vi "Detect_Level.vi"(8 "High Range":T2, 9 "Low Range":T1, 10 "EncoderDevRef":T3={"DevStatus"={"status"=FALSE, "code"=0, "source"=""}, "EncoderIndex"=enum."Invalid", "CounterIndex"=enum."Ctr 1", "DistancePerCount"=2.0, "Decoding Type"=enum."4x"}) -> (2 "Level":dbl)   [LabVIEW 2014]
uses:
  <vilib>/Rock Robotics/WPI/Encoder/WPI_EncoderDevRef.ctl
  <vilib>/Rock Robotics/SystemInterfaces/Encoder/FPGA_EncoderIdx.ctl
  <vilib>/Rock Robotics/SystemInterfaces/Counter/FPGA_CounterCtrSystemIndex.ctl
  <vilib>/Rock Robotics/WPI/Encoder/WPI_EncoderType.ctl
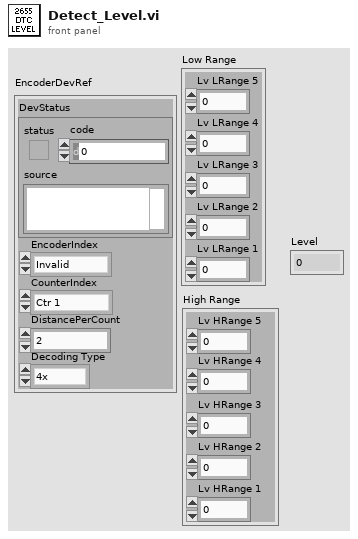
[diagram p1: front panel]
types:
  T1 = cluster{"Lv LRange 1":dbl, "Lv LRange 2":dbl, "Lv LRange 3":dbl, "Lv LRange 4":dbl, "Lv LRange 5":dbl}
  T2 = cluster{"Lv HRange 5":dbl, "Lv HRange 4":dbl, "Lv HRange 3":dbl, "Lv HRange 2":dbl, "Lv HRange 1":dbl}
  T3 = typedef "WPI_EncoderDevRef.ctl" = cluster{"DevStatus":errorcluster, "EncoderIndex":T4, "CounterIndex":T5, "DistancePerCount":dbl, "Decoding Type":T6}
  T4 = typedef "FPGA_EncoderIdx.ctl" = enum8{"Enc 0", "Enc 1", "Enc 2", "Enc 3", "Enc 4", "Enc 5", "Enc 6", "Enc 7", "Invalid"}
  T5 = typedef "FPGA_CounterCtrSystemIndex.ctl" = enum8{"Ctr 0", "Ctr 1", "Ctr 2", "Ctr 3", "Ctr 4", "Ctr 5", "Ctr 6", "Ctr 7", "Invalid"}
  T6 = typedef "WPI_EncoderType.ctl" = enum16{"1x", "2x", "4x"}
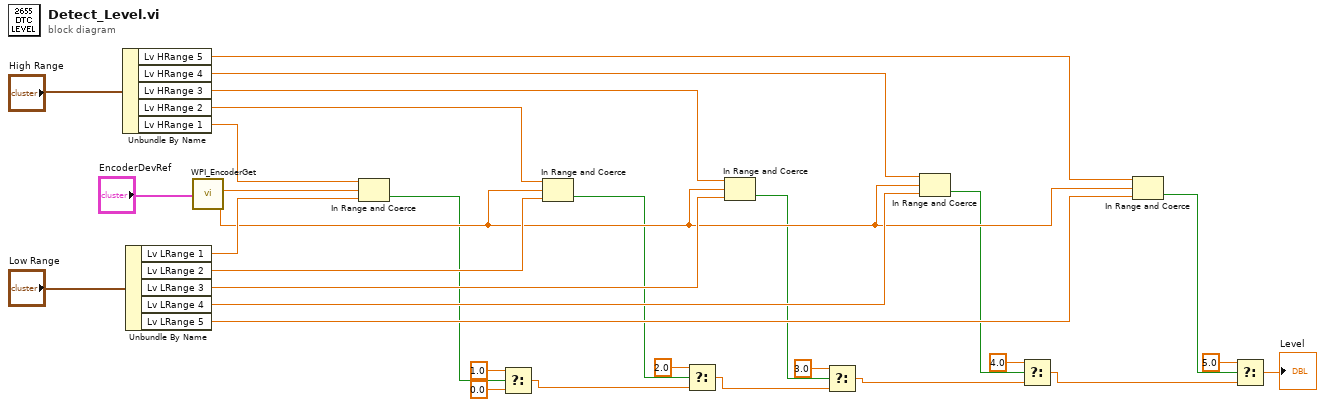
[diagram p0: block diagram]
diagram:
  n1 = Unbundle By Name("High Range") -> ("Lv HRange 5"=w18:dbl, "Lv HRange 4"=w20:dbl, "Lv HRange 3"=w23:dbl, "Lv HRange 2"=w24:dbl, "Lv HRange 1"=w26:dbl)
  n2 = Unbundle By Name("Low Range") -> ("Lv LRange 1"=w27:dbl, "Lv LRange 2"=w25:dbl, "Lv LRange 3"=w22:dbl, "Lv LRange 4"=w21:dbl, "Lv LRange 5"=w19:dbl)
  n3 = call <vilib>:"WPI_EncoderGet.vi"("EncoderDevRef"="EncoderDevRef") -> ("Distance"=w17:dbl)  [unwired: 5 in, 5 out]
  n4 = In Range and Coerce(upper limit=w26, x=w17, lower limit=w27) -> (In Range?=w16:bool)  [unwired: 1 out]
  n5 = Select(t=1.0, s=w16, f=0.0) -> (s? t:f=w6:dbl)
  n6 = In Range and Coerce(upper limit=w24, x=w17, lower limit=w25) -> (In Range?=w13:bool)  [unwired: 1 out]
  n7 = Select(t=2.0, s=w13, f=w6) -> (s? t:f=w5:dbl)
  n8 = In Range and Coerce(upper limit=w23, x=w17, lower limit=w22) -> (In Range?=w11:bool)  [unwired: 1 out]
  n9 = Select(t=3.0, s=w11, f=w5) -> (s? t:f=w4:dbl)
  n10 = In Range and Coerce(upper limit=w20, x=w17, lower limit=w21) -> (In Range?=w9:bool)  [unwired: 1 out]
  n11 = Select(t=4.0, s=w9, f=w4) -> (s? t:f=w3:dbl)
  n12 = In Range and Coerce(upper limit=w18, x=w17, lower limit=w19) -> (In Range?=w7:bool)  [unwired: 1 out]
  n13 = Select(t=5.0, s=w7, f=w3) -> (s? t:f=→"Level":dbl)
